vi "Linking Query.vi"(6 "Serial array":string[](array[string]), 9 "Parent":string, 10 "Level":u8, 11 "batch table":string) -> (3 "String":string)   [LabVIEW 2024, in "DB.lvlib"]
uses:
  DB.lvlib
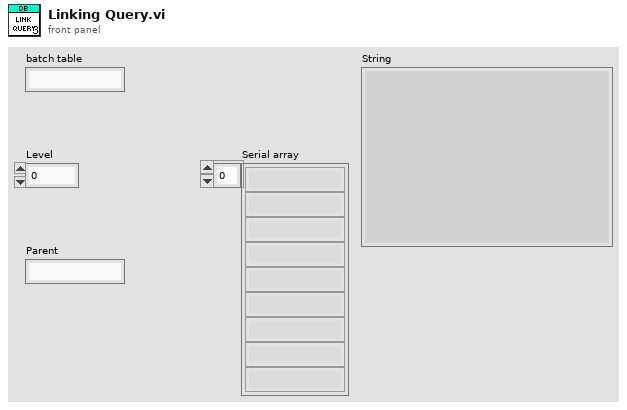
[diagram p1: front panel]
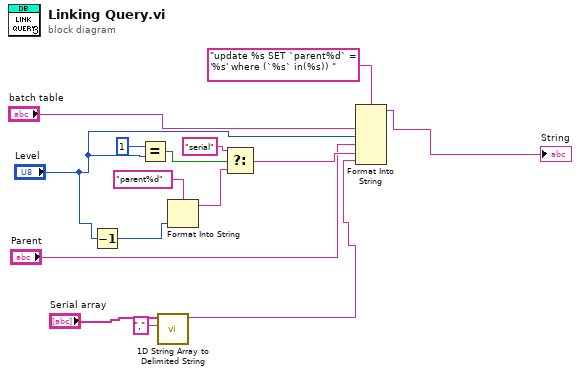
[diagram p0: block diagram]
diagram:
  n1 = Decrement(x="Level") -> (x-1=w1:u8)
  n2 = Equal?(x=u8 1, y="Level") -> (x = y?=w4:bool)
  n3 = call <vilib>:"1D String Array to Delimited String.vi"("delimiter"=",", "string array"="Serial array") -> ("delimited string"=w10:string)  [unwired: 9 in]
  n4 = Format Into String(format string="parent%d", w1) -> (resulting string=w6:string)  [unwired: 2 in, 1 out]
  n5 = Select(t="serial", s=w4, f=w6) -> (s? t:f=w14:string)
  n6 = Format Into String(format string="update %s SET `parent%d` = '%s' where (`%s` in(%s)) ", "batch table", "Level", "Parent", w14, w10) -> (resulting string=→"String":string)  [unwired: 2 in, 1 out]
